vi "Read Data as Mono14p Image.vi"(8 "error in (no error)":errorcluster, 11 "Buffer in":refnum<class "Buffer.lvclass">) -> (0 "error out":errorcluster, 2 "Image":u16[][](array[numeric]), 3 "Buffer":refnum<class "Buffer.lvclass">)   [LabVIEW 2020, in "Buffer.lvclass"]
uses:
  Buffer.lvclass
  Buffer.lvclass/Buffer.ctl
  bin/gindustrialcam_32-1.dll
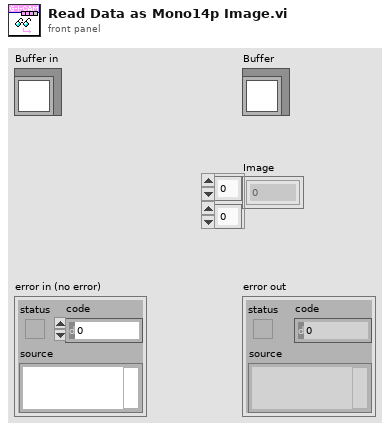
[diagram p1: front panel]
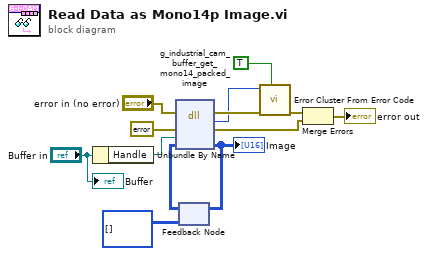
[diagram p0: block diagram]
diagram:
  n1 = Unbundle By Name("Buffer in") -> ("Handle"=w10:refnum<data-value>)
  n2 = feedback #1(u16[][] [] ("Image")) -> (w8:u16[][])
  n3 = dll-call lib="C:/serenial/lib/g-industrial-camera/LabVIEW/g_industrial_cam/bin/gindustrialcam_*-1.*" fn="g_industrial_cam_buffer_get_mono14_packed_image"(error in="error in (no error)", "err"=errorcluster {"status"=FALSE, "code"=0, "source"=""} ("error constant"), "edvr"=w10, "image"=w8) -> (error out=w7:errorcluster, "Mg_Error"=w6:i32, "err"=w4:errorcluster, "image"=w1:u16[][])  [unwired: 3 in, 1 out]
  "Image" <- w1
  n4 = feedback-in #1(w1) -> ()
  n5 = call <vilib>:"Error Cluster From Error Code.vi"("show call chain? (False)"=TRUE, "error in (no error)"=w7, "error code (0)"=w6) -> ("error out"=w5:errorcluster)  [unwired: 6 in]
  n6 = Merge Errors(w5, w4) -> (→"error out":errorcluster)
  "Buffer" <- "Buffer in"
